vi "Set Measurement_v1_MeasurementService_GetMetadata Response.vi"(7 "Streeming? (F)":bool, 8 "error in (no error)":errorcluster, 10 "Message Data":T1, 11 "gRPCid in":T7) -> (0 "error out":errorcluster)   [LabVIEW 2020, in "LoadRegulation.lvlib" / "MeasurementService_Template.lvclass"]
uses:
  MeasurementService_Template.lvclass
  <vilib>/gRPC/LabVIEW gRPC Library/Server API/typeDefs/grpcId.ctl
  RPC Messages/Measurement_v1_GetMetadataResponse/Measurement_v1_GetMetadataResponse_Data.ctl
  RPC Messages/Measurement_v1_MeasurementDetails/Measurement_v1_MeasurementDetails_Data.ctl
  RPC Messages/Measurement_v1_MeasurementParameters/Measurement_v1_MeasurementParameters_Data.ctl
  RPC Messages/Measurement_v1_ConfigurationParameter/Measurement_v1_ConfigurationParameter_Data.ctl
  RPC Messages/Measurement_v1_OutputParameter/Measurement_v1_OutputParameter_Data.ctl
  RPC Messages/Measurement_v1_UserInterfaceDetails/Measurement_v1_UserInterfaceDetails_Data.ctl
  <vilib>/gRPC/LabVIEW gRPC Library/gprc-lvsupport-release.lvlib
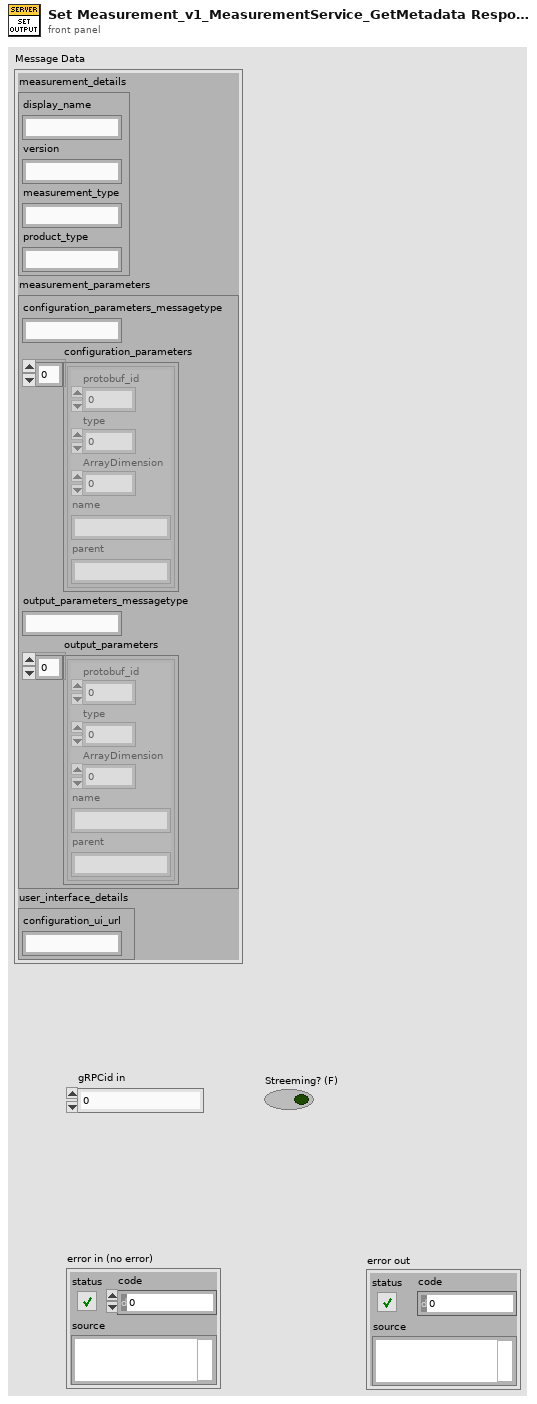
[diagram p1: front panel]
types:
  T1 = typedef "LoadRegulation.lvlib/MeasurementService_Template.lvclass/Measurement_v1_GetMetadataResponse_Data.ctl" = cluster{"measurement_details":T2, "measurement_parameters":T3, "user_interface_details":T6}
  T2 = typedef "LoadRegulation.lvlib/MeasurementService_Template.lvclass/Measurement_v1_MeasurementDetails_Data.ctl" = cluster{"display_name":string, "version":string, "measurement_type":string, "product_type":string}
  T3 = typedef "LoadRegulation.lvlib/MeasurementService_Template.lvclass/Measurement_v1_MeasurementParameters_Data.ctl" = cluster{"configuration_parameters_messagetype":string, "configuration_parameters":T4[], "output_parameters_messagetype":string, "output_parameters":T5[]}
  T4 = typedef "LoadRegulation.lvlib/MeasurementService_Template.lvclass/Measurement_v1_ConfigurationParameter_Data.ctl" = cluster{"protobuf_id":i32, "type":i32, "ArrayDimension":i32, "name":string, "parent":string}
  T5 = typedef "LoadRegulation.lvlib/MeasurementService_Template.lvclass/Measurement_v1_OutputParameter_Data.ctl" = cluster{"protobuf_id":i32, "type":i32, "ArrayDimension":i32, "name":string, "parent":string}
  T6 = typedef "LoadRegulation.lvlib/MeasurementService_Template.lvclass/Measurement_v1_UserInterfaceDetails_Data.ctl" = cluster{"configuration_ui_url":string}
  T7 = typedef "gprc-lvsupport-release.lvlib/grpcId.ctl" = u64
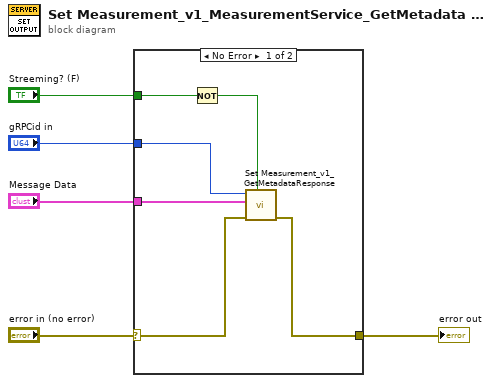
[diagram p0: block diagram]
diagram:
  n1 = case shown="No Error" "error in (no error)" {
    selector: "error in (no error)" -> [w11 w12]
    tunnel: [w9 w12] -> w4
    tunnel: "gRPCid in" -> [w10 _]
    tunnel: "Message Data" -> [w8 _]
    tunnel: "Streeming? (F)" -> [w7 _]
    frame No Error {
      n2 = Not(x=w7) -> (.not. x?=w6:bool)
      n3 = call "Set Measurement_v1_GetMetadataResponse.vi"("Complete Call (T)"=w6, "error in (no error)"=w11, "Message Data"=w8, "gRPCid"=w10) -> ("error out"=w9:errorcluster)  [unwired: 7 in]
    }
    frame Error {
    }
  }
  "error out" <- w4
